vi "Error_LogToFile.vi"(8 "error in":errorcluster, 11 "path":path) -> (0 "error out":errorcluster)   [LabVIEW 2022 SP3, in "hse-misc.lvlib"]
doc: "If <b>error in</b> is true, writes the error to the file identified by <b>path</b> and clears the error.\n\n\n\n____\nHAMPEL SOFTWARE ENGINEERING v3.8.0 (2023-12-18 14:41)"
uses:
  hse-misc.lvlib
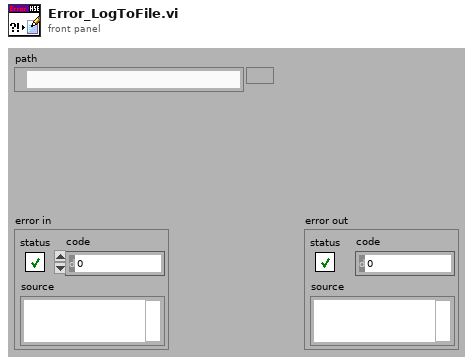
[diagram p1: front panel]
types:
  T1 = enum16{"open", "replace", "create", "open or create", "replace or create", "replace or create with confirmation"}
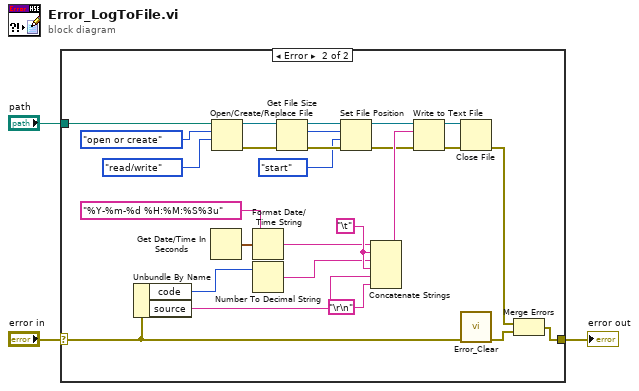
[diagram p0: block diagram]
diagram:
  n1 = case shown="Error" "error in" {
    selector: "error in" -> [w4 w29]
    tunnel: [w4 w12] -> w3
    tunnel: "path" -> [_ w25]
    frame No Error {
    }
    frame Error {
      w9 = "\t"
      n2 = Unbundle By Name(w29) -> ("code"=w24:i32, "source"=w8:string)
      n3 = Get Date/Time In Seconds() -> (seconds since 1Jan1904=w23:timestamp)
      n4 = Open/Create/Replace File(file path (use dialog)=w25, operation (0:open)=T1."open or create", access (0:read/write)=enum16{"read/write", "read-only", "write-only"}."read/write") -> (refnum out=w19:refnum<file>, error out=w18:errorcluster)  [unwired: 3 in, 1 out]
      n5 = Format Date/Time String(time format string (%c)="%Y-%m-%d %H:%M:%S%3u", seconds (now)=w23) -> (date/time string=w5:string)  [unwired: 1 out]
      n6 = Number To Decimal String(number=w24) -> (decimal integer string=w7:string)  [unwired: 1 out]
      n7 = Get File Size(file=w19, error in=w18) -> (refnum out=w21:refnum<file>, size (in bytes)=w20:i64, 0:w15:errorcluster)
      n8 = Set File Position(offset (in bytes) (0)=w20, refnum=w21, from (0:start)=enum16{"start", "end", "current"}."start", error in=w15) -> (refnum out=w17:refnum<file>, error out=w16:errorcluster)
      n9 = Concatenate Strings(w5, w9, w7, w9, w8, "\r\n") -> (w28:string)
      n10 = Write to Text File(file (use dialog)=w17, text=w28, error in=w16) -> (refnum out=w27:refnum<file>, error out=w26:errorcluster)  [unwired: 2 out]
      n11 = Close File(refnum=w27, error in=w26) -> (error out=w14:errorcluster)  [unwired: 1 out]
      n12 = call "Error_Clear.vi"("error in"=w29) -> ("error out (no error)"=w13:errorcluster)  [unwired: 10 in]
      n13 = Merge Errors(w14, w13) -> (w12:errorcluster)
    }
  }
  "error out" <- w3
